vi "Close Adu Device.vi"(8 "error in (no error)":errorcluster, 11 "Device Handle":u32) -> (0 "error out":errorcluster)   [LabVIEW 2015, in "AduHid.lvlib"]
doc: "void __stdcall CloseAduDevice(void * hDevice);"
uses:
  AduHid.lvlib
  AduHid.dll
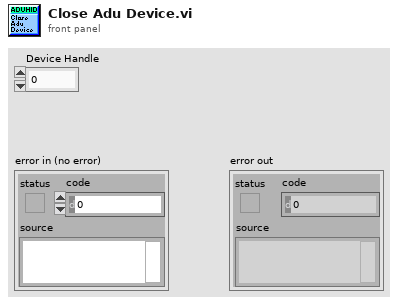
[diagram p1: front panel]
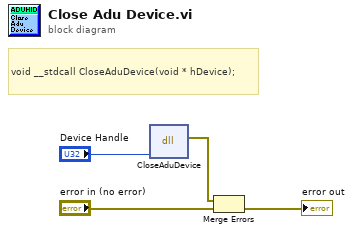
[diagram p0: block diagram]
diagram:
  # "void __stdcall CloseAduDevice(void * hDevice);"
  n1 = dll-call lib="C:/Projects/CBTF Modules/Libraries/Ontrak ADU/API/AduHid.*" fn="CloseAduDevice"("Device Handle"="Device Handle") -> (error out=w1:errorcluster)  [unwired: 5 in, 1 out]
  n2 = Merge Errors(w1, "error in (no error)") -> (→"error out":errorcluster)
